vi "refresh illumination stuff.vi"(8 "error in (no error)":errorcluster, 11 "Waveform in":refnum<class "Waveform.lvclass">) -> (0 "error out":errorcluster, 3 "Waveform out":refnum<class "Waveform.lvclass">)   [LabVIEW 2012, in "Waveform.lvclass"]
uses:
  Waveform.lvclass
  Waveform.lvclass/Waveform.ctl
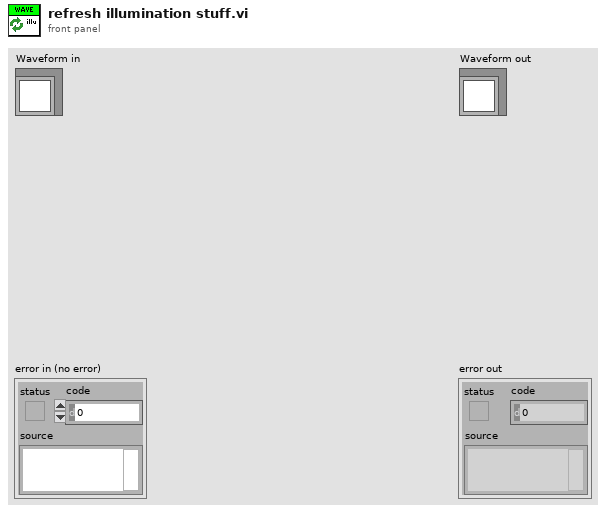
[diagram p1: front panel]
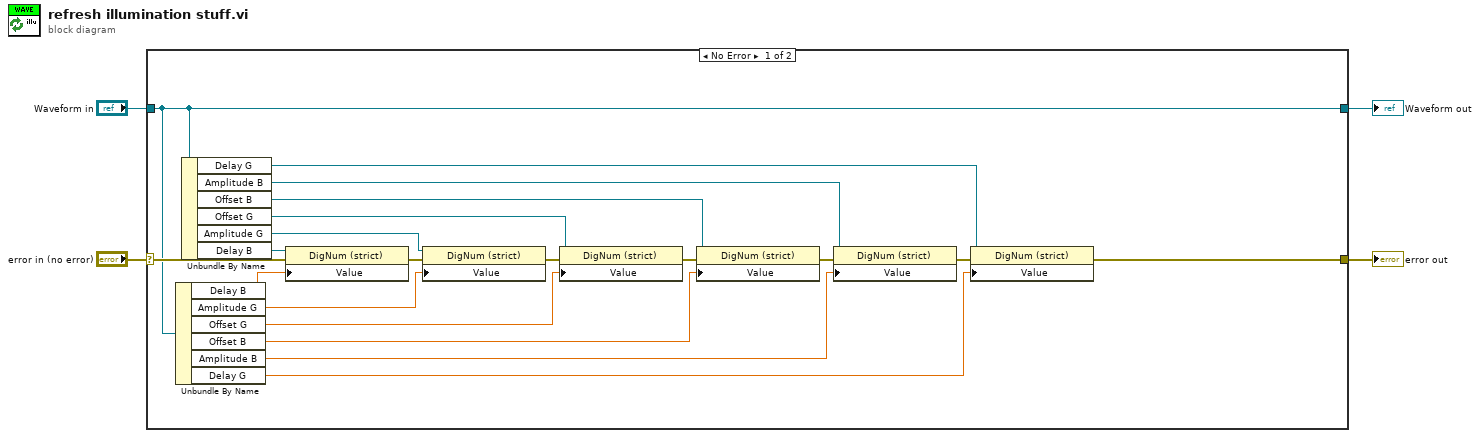
[diagram p0: block diagram]
diagram:
  n1 = case shown="No Error" "error in (no error)" {
    selector: "error in (no error)" -> [w13 w26]
    tunnel: [w5 w26] -> w3
    tunnel: [w12 w25] -> w1
    tunnel: "Waveform in" -> [w12 w25]
    frame No Error {
      n2 = Unbundle By Name(w12) -> ("Delay B"=w11:dbl[unit], "Amplitude G"=w10:dbl[unit], "Offset G"=w9:dbl[unit], "Offset B"=w8:dbl[unit], "Amplitude B"=w7:dbl[unit], "Delay G"=w6:dbl[unit])
      n3 = Unbundle By Name(w12) -> ("Delay G"=w14:refnum<vi>, "Amplitude B"=w15:refnum<vi>, "Offset B"=w16:refnum<vi>, "Offset G"=w17:refnum<vi>, "Amplitude G"=w18:refnum<vi>, "Delay B"=w24:refnum<vi>)
      n4 = property class="DigNum (strict)"(reference=w24, error in=w13, "Value"=w11) -> (error out=w22:errorcluster)  [unwired: 1 out]
      n5 = property class="DigNum (strict)"(reference=w18, error in=w22, "Value"=w10) -> (error out=w23:errorcluster)  [unwired: 1 out]
      n6 = property class="DigNum (strict)"(reference=w17, error in=w23, "Value"=w9) -> (error out=w21:errorcluster)  [unwired: 1 out]
      n7 = property class="DigNum (strict)"(reference=w16, error in=w21, "Value"=w8) -> (error out=w20:errorcluster)  [unwired: 1 out]
      n8 = property class="DigNum (strict)"(reference=w15, error in=w20, "Value"=w7) -> (error out=w19:errorcluster)  [unwired: 1 out]
      n9 = property class="DigNum (strict)"(reference=w14, error in=w19, "Value"=w6) -> (error out=w5:errorcluster)  [unwired: 1 out]
    }
    frame Error {
    }
  }
  "error out" <- w3
  "Waveform out" <- w1
